vi "PathPlanner_WPITrajHolPose_Sample.vi"(9 "Time":dbl, 11 "WPIHolonomicPose":T4[](array[typedef]) {"HolonomicPose"."ROTATION"."SIN" format="%13.4f"; "HolonomicPose"."ROTATION"."COS" format="%13.4f"; "HolonomicPose"."ROTATION"."VALUE" format="%13.4f"; "HolonomicPose"."TRANSLATION"."Y" format="%14.3f"; "HolonomicPose"."TRANSLATION"."X" format="%14.3f"}) -> (3 "HolonomicPose":T1={"TRANSLATION"={"X"=0.0, "Y"=0.0}, "ROTATION"={"VALUE"=0.0, "COS"=1.0, "SIN"=0.0}} {"ROTATION"."SIN" format="%13.4f"; "ROTATION"."COS" format="%13.4f"; "ROTATION"."VALUE" format="%13.4f"; "TRANSLATION"."Y" format="%14.3f"; "TRANSLATION"."X" format="%14.3f"})   [LabVIEW 2019, in "PathPlanner24.lvlib"]
doc: "Sample the WPI Trajectory Holonomic Pose array at a point in time\n\nInputs:\n -- WPIHolonomicPose - array - WPI Holonomic Pose data cluster\n -- time -- The time to sample\n\nOutputs:\n - HolonomicPose - pose2d - Desired holonomic pose at the given time."
uses:
  PathPlanner24.lvlib
  TypeDef/PathPlannerWPITrajHolonomicPose.ctl
  <vilib>/Rock Robotics/WPI/ThirdParty/JAS_Junk/TrajLib/TypeDef/POSE2D.ctl
  <vilib>/Rock Robotics/WPI/ThirdParty/JAS_Junk/TrajLib/TypeDef/TRANSLATION2D.ctl
  <vilib>/Rock Robotics/WPI/ThirdParty/JAS_Junk/TrajLib/TypeDef/ROTATION2D.ctl
  <vilib>/Rock Robotics/WPI/ThirdParty/JAS_Junk/TrajLib/Twist2d_GetAll.vi
  <vilib>/Rock Robotics/WPI/ThirdParty/JAS_Junk/TrajLib/Twist2d_Create.vi
  <vilib>/Rock Robotics/WPI/ThirdParty/JAS_Junk/TrajLib/Pose2d_Log.vi
  <vilib>/Rock Robotics/WPI/ThirdParty/JAS_Junk/TrajLib/Pose2d_Exp.vi
  <vilib>/Rock Robotics/WPI/ThirdParty/JAS_Junk/TrajLib/Trajectory_Library.lvlib
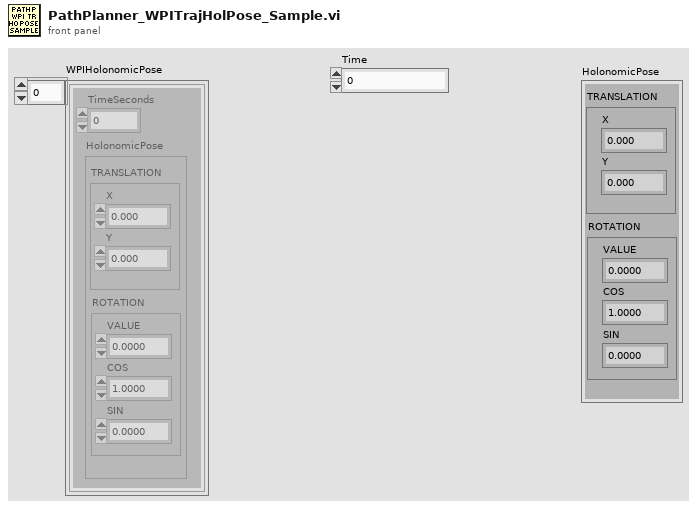
[diagram p1: front panel]
types:
  T1 = typedef "Trajectory_Library.lvlib/POSE2D.ctl" = cluster{"TRANSLATION":T2, "ROTATION":T3}
  T2 = typedef "Trajectory_Library.lvlib/TRANSLATION2D.ctl" = cluster{"X":dbl, "Y":dbl}
  T3 = typedef "Trajectory_Library.lvlib/ROTATION2D.ctl" = cluster{"VALUE":dbl, "COS":dbl, "SIN":dbl}
  T4 = typedef "PathPlanner24.lvlib/PathPlannerWPITrajHolonomicPose.ctl" = cluster{"TimeSeconds":dbl, "HolonomicPose":T1}
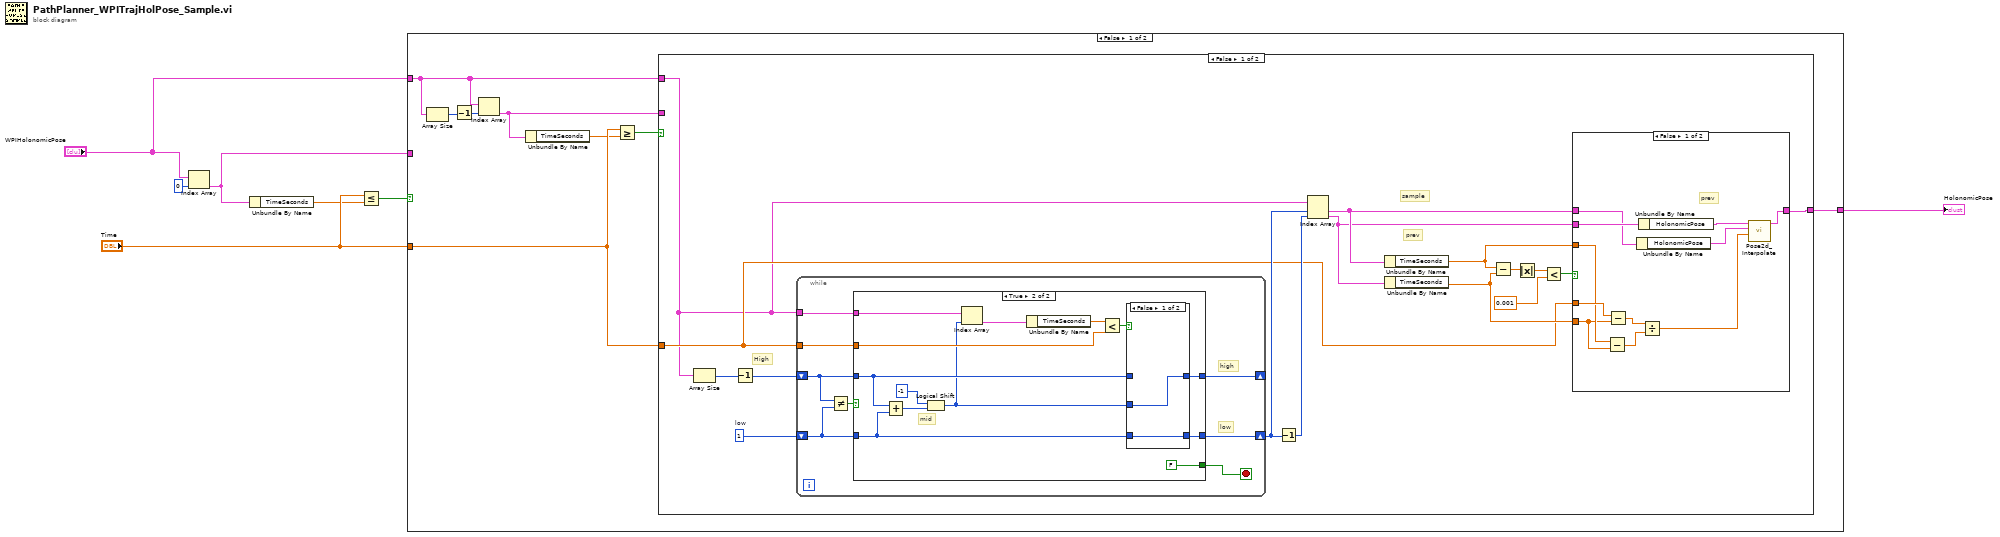
[diagram p0: block diagram]
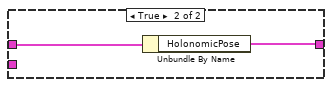
[diagram p2: hidden frame]
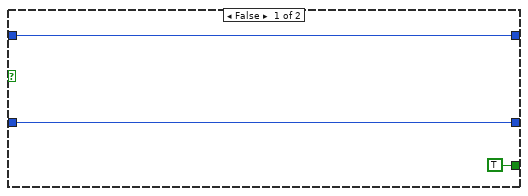
[diagram p3: hidden frame]
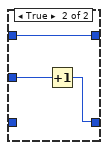
[diagram p4: hidden frame]
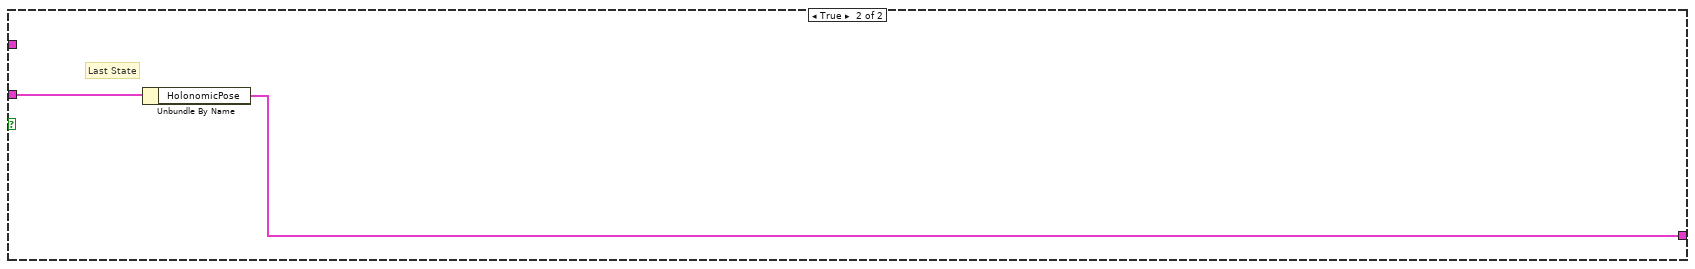
[diagram p5: hidden frame]
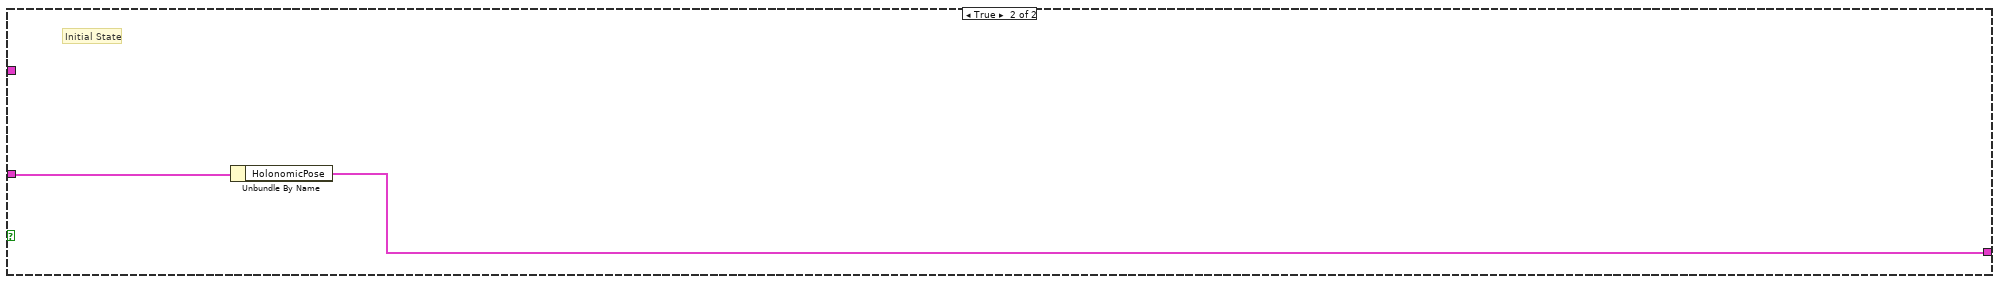
[diagram p6: hidden frame]
diagram:
  n1 = Index Array(array="WPIHolonomicPose", index=0) -> (element=w3:T4)
  n2 = Unbundle By Name(w3) -> ("TimeSeconds"=w4:dbl)
  n3 = Less Or Equal?(x="Time", y=w4) -> (x <= y?=w7:bool)
  n4 = case shown="False" w7 {
    tunnel: [w14 w76] -> w2
    tunnel: "WPIHolonomicPose" -> [w10 _]
    tunnel: "Time" -> [w13 _]
    tunnel: w3 -> [_ w77]
    frame False {
      n5 = Array Size(array=w10) -> (size(s)=w12:i32)
      n6 = Decrement(x=w12) -> (x-1=w11:i32)
      n7 = Index Array(array=w10, index=w11) -> (element=w8:T4)
      n8 = Unbundle By Name(w8) -> ("TimeSeconds"=w9:dbl)
      n9 = Greater Or Equal?(x=w13, y=w9) -> (x >= y?=w15:bool)
      n10 = case shown="False" w15 {
        tunnel: [w21 w74] -> w14
        tunnel: w10 -> [w16 _]
        tunnel: w13 -> [w18 _]
        tunnel: w8 -> [_ w75]
        frame False {
          w29 = 1  # low
          # "prev"
          # "sample"
          # "High"
          n11 = Array Size(array=w16) -> (size(s)=w31:i32)
          n12 = Decrement(x=w31) -> (x-1=w30:i32)
          n13 = while {
            shift-right: [w50] -> w28
            shift-left: w29 -> [w46]
            shift-right: [w51] -> _
            shift-left: w30 -> [w47]
            tunnel: w16 -> [w49]
            tunnel: w18 -> [w52]
            stop <- w45 stop-if-true
            # "high"
            # "low"
            n14 = Not Equal?(x=w47, y=w46) -> (x != y?=w48:bool)
            n15 = case shown="True" w48 {
              tunnel: w52 -> [_ w65]
              tunnel: w47 -> [w55 w63]
              tunnel: w46 -> [w54 w62]
              tunnel: [w55 w61] -> w51
              tunnel: [w54 w60] -> w50
              tunnel: w49 -> [_ w58]
              tunnel: [TRUE FALSE] -> w45
              frame False {
              }
              frame True {
                # "mid"
                n16 = Add(x=w63, y=w62) -> (x+y=w68:i32)
                n17 = Logical Shift(y=i16 -1, x=w68) -> (x << y=w57:i32)
                n18 = Index Array(array=w58, index=w57) -> (element=w56:T4)
                n19 = Unbundle By Name(w56) -> ("TimeSeconds"=w66:dbl)
                n20 = Less?(x=w66, y=w65) -> (x < y?=w64:bool)
                n21 = case shown="False" w64 {
                  tunnel: w63 -> [_ w73]
                  tunnel: [w69 w73] -> w61
                  tunnel: w57 -> [w69 w72]
                  tunnel: w62 -> [w70 _]
                  tunnel: [w70 w71] -> w60
                  frame False {
                  }
                  frame True {
                    n22 = Increment(x=w72) -> (x+1=w71:i32)
                  }
                }
              }
            }
          }
          n23 = Decrement(x=w28) -> (x-1=w27:i32)
          n24 = Index Array(array=w16, index #1=w28, index #2=w27) -> (element #1=w22:T4, element #2=w20:T4)
          n25 = Unbundle By Name(w22) -> ("TimeSeconds"=w17:dbl)
          n26 = Unbundle By Name(w20) -> ("TimeSeconds"=w19:dbl)
          n27 = Subtract(x=w17, y=w19) -> (x-y=w26:dbl)
          n28 = Absolute Value(x=w26) -> (abs(x)=w25:dbl)
          n29 = Less?(x=w25, y=0.001) -> (x < y?=w23:bool)
          n30 = case shown="False" w23 {
            tunnel: w22 -> [w35 w44]
            tunnel: [w32 w43] -> w21
            tunnel: w20 -> [w37 _]
            tunnel: w19 -> [w40 _]
            tunnel: w18 -> [w42 _]
            tunnel: w17 -> [w41 _]
            frame False {
              # "prev"
              n31 = Subtract(x=w41, y=w40) -> (x-y=w38:dbl)
              n32 = Subtract(x=w42, y=w40) -> (x-y=w39:dbl)
              n33 = Unbundle By Name(w35) -> ("HolonomicPose"=w34:T1)
              n34 = Unbundle By Name(w37) -> ("HolonomicPose"=w36:T1)
              n35 = Divide(x=w39, y=w38) -> (x/y=w33:dbl)
              n36 = call <vilib>:"Pose2d_Interpolate.vi"("T"=w33, "EndValue Pose"=w34, "in POSE"=w36) -> ("Interpolated Pose"=w32:T1)  [unwired: 8 in]
            }
            frame True {
              n37 = Unbundle By Name(w44) -> ("HolonomicPose"=w43:T1)
            }
          }
        }
        frame True {
          # "Last State"
          n38 = Unbundle By Name(w75) -> ("HolonomicPose"=w74:T1)
        }
      }
    }
    frame True {
      # "Initial State"
      n39 = Unbundle By Name(w77) -> ("HolonomicPose"=w76:T1)
    }
  }
  "HolonomicPose" <- w2
